vi "m1m3_acceptCommand_ApplyActiveOpticForcesByBendingModes.vi"(8 "error in (no error)":errorcluster, 11 "command_ApplyActiveOpticForcesByBendingModes_Ctl":T1={"Coefficients[22]"=[0.0, 0.0, 0.0, 0.0, 0.0, 0.0, 0.0, 0.0, 0.0, 0.0, 0.0, 0.0, 0.0, 0.0, 0.0, 0.0, 0.0, 0.0, 0.0, 0.0, 0.0, 0.0]}) -> (0 "error out":errorcluster, 2 "function return":i32, 3 "command_ApplyActiveOpticForcesByBendingModes_Ctl out":T1)   [LabVIEW 2016, in "SALLV_m1m3.lvlib"]
doc: "int m1m3_shm_acceptCommand_ApplyActiveOpticForcesByBendingModesLV(m1m3_command_ApplyActiveOpticForcesByBendingModesLV *command_ApplyActiveOpticForcesByBendingModes_Ctl );"
uses:
  SALLV_m1m3.lvlib
  DataTypes/command_ApplyActiveOpticForcesByBendingModes.ctl
  SALLV_m1m3.so
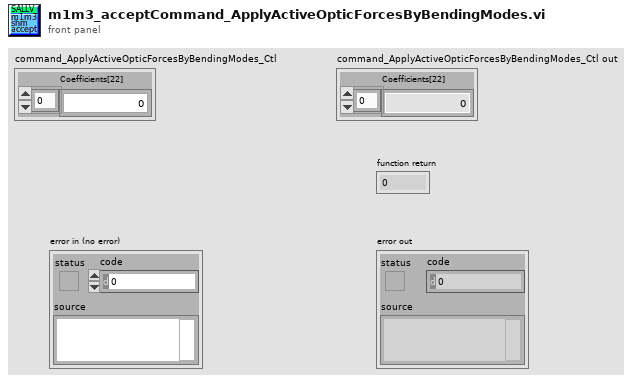
[diagram p1: front panel]
types:
  T1 = typedef "SALLV_m1m3.lvlib/command_ApplyActiveOpticForcesByBendingModes.ctl" = cluster{"Coefficients[22]":sgl[]}
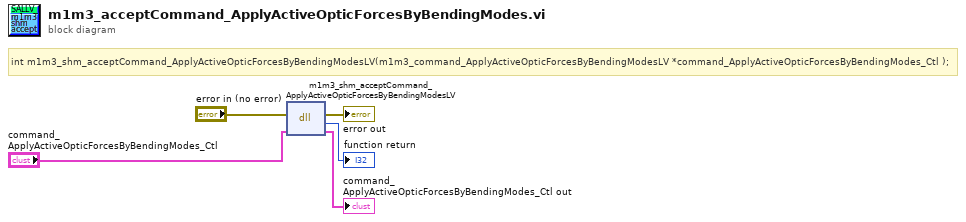
[diagram p0: block diagram]
diagram:
  # "int m1m3_shm_acceptCommand_ApplyActiveOpticForcesByBendingModesLV(m1m3_command_ApplyActiveOpticForcesByBendingModesLV *command_ApplyActiveOpticForcesByBendingModes_Ctl );"
  n1 = dll-call lib="opt/CODE/SALLV_m1m3/SALLV_m1m3.*" fn="m1m3_shm_acceptCommand_ApplyActiveOpticForcesByBendingModesLV"(error in="error in (no error)", "command_ApplyActiveOpticForcesByBendingModes_Ctl"="command_ApplyActiveOpticForcesByBendingModes_Ctl") -> (error out=→"error out":errorcluster, →"function return":i32, "command_ApplyActiveOpticForcesByBendingModes_Ctl"=→"command_ApplyActiveOpticForcesByBendingModes_Ctl out":T1)  [unwired: 2 in, 1 out]
